vi "ErrorManager.vi"(3 "error in (no error)":errorcluster {"code" format="%x"}, 5 "error code":i32 format="%x") -> (0 "error out":errorcluster {"code" format="%x"}, 1 "statusWarning":bool)   [LabVIEW 2019]
doc: "ErrorManager tranlsates error numbers generated by the pco.camera interface into language. Information on the source of the error, the device and software layer where the error originated is coded into the error string. \nThis function is called by all SDK and recorder SDK functions, so that error numbers can be converted into LabVIEW error clusters for further handling."
panel:
  out "statusError":bool
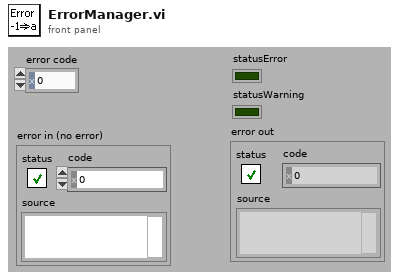
[diagram p1: front panel]
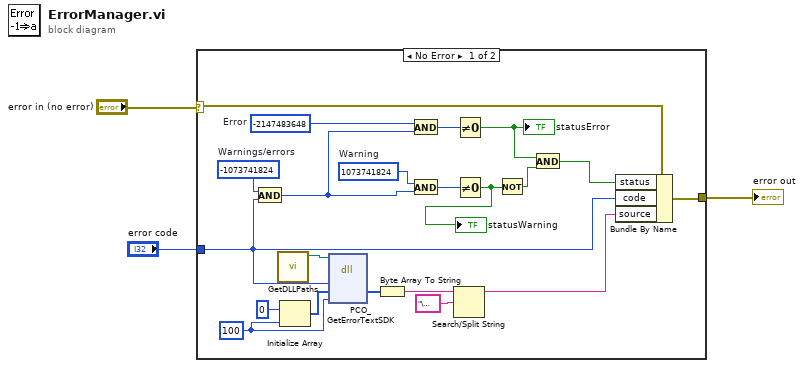
[diagram p0: block diagram]
diagram:
  n1 = case shown="No Error" "error in (no error)" {
    selector: "error in (no error)" -> [w15 w25]
    tunnel: [w17 w25] -> w1
    tunnel: "error code" -> [w12 _]
    frame No Error {
      w7 = 1073741824  # Warning
      w13 = -2147483648  # Error
      w14 = -1073741824  # Warnings/errors
      w22 = u32 100 ("dimension size")
      n2 = And(x=w14, y=w12) -> (x .and. y?=w8:i32)
      n3 = call "GetDLLPaths.vi"() -> ("SC2_Cam_Path"=w16:path)  [unwired: 8 in, 3 out]
      n4 = Initialize Array(u8 0, w22) -> (w23:u8[])
      n5 = dll-call lib="?" fn="PCO_GetErrorTextSDK"(path in=w16, "errorCode"=w12, "pBuf"=w23, "bufLength"=w22) -> ("pBuf"=w20:u8[])  [unwired: 5 in, 2 out]
      n6 = Byte Array To String(unsigned byte array=w20) -> (string=w21:string)
      n7 = And(x=w13, y=w8) -> (x .and. y?=w11:i32)
      n8 = And(x=w7, y=w8) -> (x .and. y?=w9:i32)
      n9 = Search/Split String(string=w21, search string/char (-)="\u0000" ("search string")) -> (substring before match=w18:string)  [unwired: 1 in, 2 out]
      n10 = Not Equal To 0?(x=w11) -> (x != 0?=w10:bool)
      "statusError" <- w10
      n11 = Not Equal To 0?(x=w9) -> (x != 0?=w5:bool)
      "statusWarning" <- w5
      n12 = Not(x=w5) -> (.not. x?=w4:bool)
      n13 = And(x=w10, y=w4) -> (x .and. y?=w6:bool)
      n14 = Bundle By Name(cluster=w15, "status"=w6, "code"=w12, "source"=w18) -> (w17:errorcluster)
    }
    frame Error {
    }
  }
  "error out" <- w1
